vi "Do Request.vi"(7 "Processing In":refnum<class "Processing.lvclass">, 11 "Submission API in":refnum<class "User Submissions API.lvclass">) -> (0 "error out":errorcluster, 5 "Processing":refnum<class "Processing.lvclass">)   [LabVIEW 2020, in "Summer of LabVIEW.lvlib" / "User Submissions API.lvclass"]
uses:
  User Submissions API.lvclass
  <vilib>/IlluminatedG/IG HTTP Server/HTTP Server/Processing/Processing.lvclass
  Submission DB/Submission DB.lvclass
  SOL User/SOL User.lvclass
  <vilib>/IlluminatedG/IG HTTP Server/HTTP Server/Processing/Processing.lvclass/Processing.ctl
  Data Types/Submission JSON.ctl
  SoL Scoring/Score.ctl
  SoL Scoring/Score Entry.ctl
  13ece07f-56c7-4085-a057-43fbaccaa13e.vi
  d6c464f8-b06b-4d93-b557-cc6d28ba9314.vi
  f9cb6381-3961-4b78-a24d-5306bd3c4dd1.vi
  13ece07f-56c7-4085-a057-43fbaccaa13e.vi/36b1f833-cfc6-44a5-864d-b53e3b32e5c8.vi
  d6c464f8-b06b-4d93-b557-cc6d28ba9314.vi/9528e9df-aefc-4ce0-9221-106a337fd3b6.vi
  f9cb6381-3961-4b78-a24d-5306bd3c4dd1.vi/9528e9df-aefc-4ce0-9221-106a337fd3b6.vi
  <vilib>/IlluminatedG/IG HTTP Server/HTTP Server/Values/Get Arg Map.vi
  <vilib>/Utility/error.llb/Error Cluster From Error Code.vi
  User Submissions API.lvclass/User Submissions API.ctl
  SoL Scoring/SoL Scoring.lvlib
  Summer of LabVIEW.lvlib
  <vilib>/IlluminatedG/IG HTTP Utils/HTTP Utils/Response/Response.lvclass
  Submission/Submission.lvclass
  <vilib>/IlluminatedG/lv-web-crypto/lv-json/JSON/JSON.lvlib
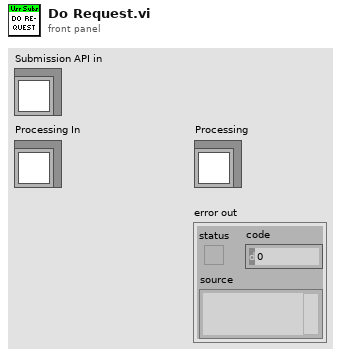
[diagram p1: front panel]
types:
  T1 = typedef "Summer of LabVIEW.lvlib/Submission JSON.ctl" = cluster{"ID":i64, "Submitted":string, "Score":T2, "Tested":bool, "Test_Timestamp":string, "Test_Summary":string}
  T2 = typedef "SoL Scoring.lvlib/Score.ctl" = cluster{"Overall":dbl, "Categories":T3[]}
  T3 = typedef "SoL Scoring.lvlib/Score Entry.ctl" = cluster{"Category":string, "Value":dbl}
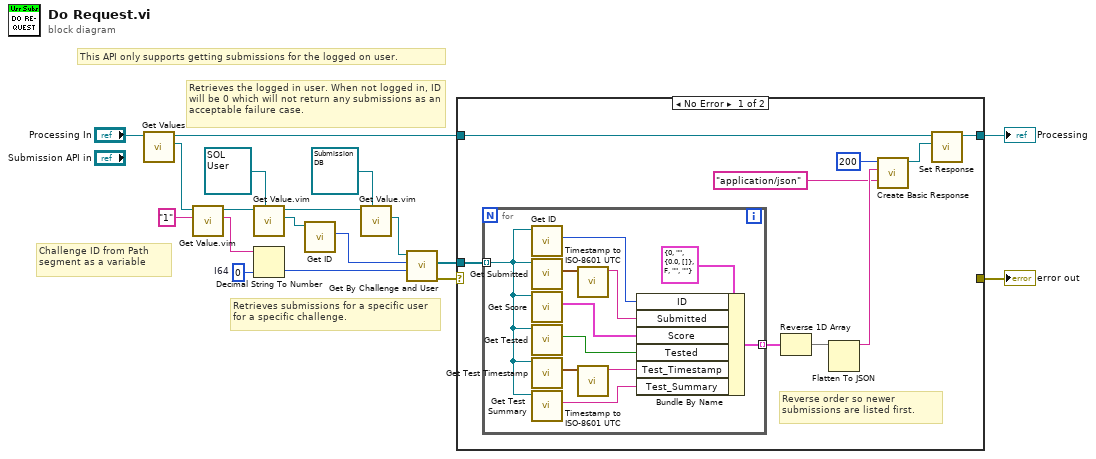
[diagram p0: block diagram]
diagram:
  w14 = i64 0  # I64
  # "Retrieves submissions for a specific user for a specific challenge."
  # "Retrieves the logged in user. When not logged in, ID will be 0 which will not return any submissions as an acceptable failure case."
  # "Challenge ID from Path segment as a variable"
  # "This API only supports getting submissions for the logged on user."
  n1 = call <vilib>:"Get Values.vi"("Processing in"="Processing In") -> ("Values"=w17:refnum<class "Values.lvclass">, "Processing out"=w10:refnum<class "Processing.lvclass">)  [unwired: 9 in]
  n2 = call "Get Value.vim"("Name for Type"="1", "Arguments in"=w17) -> ("Value"=w15:string, "Arguments out"=w9:refnum<class "Values.lvclass">)  [unwired: 7 in, 1 out]
  n3 = call "Get Value.vim"("Type / Server / Service (String)"=refnum<class "SOL User.lvclass"> refnum ("SOL:SOL User.lvclass"), "Arguments in"=w9) -> ("Value"=w11:refnum<class "SOL User.lvclass">, "Arguments out"=w8:refnum<class "Values.lvclass">)  [unwired: 7 in, 1 out]
  n4 = Decimal String To Number(string=w15, default (0L)=w14) -> (number=w5:i64)  [unwired: 1 in, 1 out]
  n5 = call "Get ID.vi"("SOL User in"=w11) -> ("ID"=w6:i64)  [unwired: 8 in, 2 out]
  n6 = call "Get Value.vim"("Type / Server / Service (String)"=refnum<class "Submission DB.lvclass"> refnum ("SOL:Submission DB.lvclass"), "Arguments in"=w8) -> ("Value"=w7:refnum<class "Submission DB.lvclass">)  [unwired: 7 in, 2 out]
  n7 = call "Get By Challenge and User.vi"("Challenge ID"=w5, "User ID"=w6, "Submission DB in"=w7) -> ("error out"=w4:errorcluster, "Submissions"=w3:refnum<class "Submission.lvclass">[])  [unwired: 6 in, 1 out]
  n8 = case shown="No Error" w4 {
    selector: w4 -> [_ w39]
    tunnel: w10 -> [w22 w40]
    tunnel: w3 -> [w27 _]
    tunnel: [w20 w40] -> w2
    tunnel: [_ w39] -> w1
    frame No Error {
      # "Reverse order so newer submissions are listed first."
      n9 = for {
        tunnel: w27 -> [w29] mode=indexing
        tunnel: [w37] -> w26 mode=indexing
        n10 = call "Get ID.vi"("Submission in"=w29) -> ("ID"=w36:i64)  [unwired: 9 in, 1 out]
        n11 = call "Get Submitted.vi"("Submission in"=w29) -> ("Submitted"=w35:timestamp)  [unwired: 9 in, 1 out]
        n12 = call "Get Score.vi"("Submission in"=w29) -> ("Score"=w33:T2)  [unwired: 9 in, 1 out]
        n13 = call "Get Tested.vi"("Submission in"=w29) -> ("Tested"=w32:bool)  [unwired: 9 in, 1 out]
        n14 = call "Get Test Timestamp.vi"("Submission in"=w29) -> ("Test Timestamp"=w30:timestamp)  [unwired: 9 in, 1 out]
        n15 = call "Get Test Summary.vi"("Submission in"=w29) -> ("Test Summary"=w28:string)  [unwired: 9 in, 1 out]
        n16 = call <vilib>:"Timestamp to ISO-8601 UTC.vi"("Time Stamp"=w35) -> ("ISO 8601 UTC"=w34:string)  [unwired: 10 in]
        n17 = call <vilib>:"Timestamp to ISO-8601 UTC.vi"("Time Stamp"=w30) -> ("ISO 8601 UTC"=w31:string)  [unwired: 10 in]
        n18 = Bundle By Name(cluster=T1 {"ID"=0, "Submitted"="", "Score"={"Overall"=0.0, "Categories"=[]}, "Tested"=FALSE, "Test_Timestamp"="", "Test_Summary"=""} ("Submission JSON"), "ID"=w36, "Submitted"=w34, "Score"=w33, "Tested"=w32, "Test_Timestamp"=w31, "Test_Summary"=w28) -> (w37:T1)
      }
      n19 = Reverse 1D Array(array=w26) -> (reversed array=w19:T1[])
      n20 = Flatten To JSON(anything=w19) -> (JSON string=w24:string)  [unwired: 2 in, 1 out]
      n21 = call <vilib>:"Create Basic Response.vi"("Content-Type (text/plain)"="application/json", "Payload"=w24, "Status Code"=u16 200) -> ("Response out"=w21:refnum<class "Response.lvclass">)  [unwired: 7 in, 1 out]
      n22 = call <vilib>:"Set Response.vi"("Response"=w21, "Processing in"=w22) -> ("Processing out"=w20:refnum<class "Processing.lvclass">)  [unwired: 9 in]
    }
    frame Error {
      # "Let the error pass out which will generally return a 500 status to the client."
    }
  }
  "error out" <- w1
  "Processing" <- w2
